vi "Remove Sink.vi"(8 "error in (no error)":errorcluster, 9 "Remove All (F)":bool, 10 "Sink Name":string, 11 "Event Source in":refnum<class "Event Source.lvclass">) -> (0 "error out":errorcluster, 3 "Event Source out":refnum<class "Event Source.lvclass">)   [LabVIEW 2016, in "Event Source.lvlib" / "Event Source.lvclass"]
doc: "Stops and removes a sink actor as specified by his name. Can remove all the sinks if the \"Remove All (F)\" is set to true"
uses:
  Event Source.lvclass
  Event Source.lvclass/Event Source.ctl
  Sink Details.ctl
  <vilib>/ActorFramework/Message Enqueuer/Message Enqueuer.lvclass
  <vilib>/ActorFramework/Message Enqueuer/Message Enqueuer.lvclass/Message Enqueuer.ctl
  <vilib>/ActorFramework/Message Enqueuer/Enqueue.vi
  <vilib>/ActorFramework/Stop Msg/Stop Msg.lvclass
  C:/Program Files (x86)/National Instruments/LabVIEW 2016/vi.lib/ActorFramework/Message/Message.lvclass
  <vilib>/Utility/LVClass/Get LV Class Name.vi
  <resource>/AFDebug/Generate Trace for Message.vi
  <vilib>/ActorFramework/Message Priority Queue/Priority Enqueue.vi
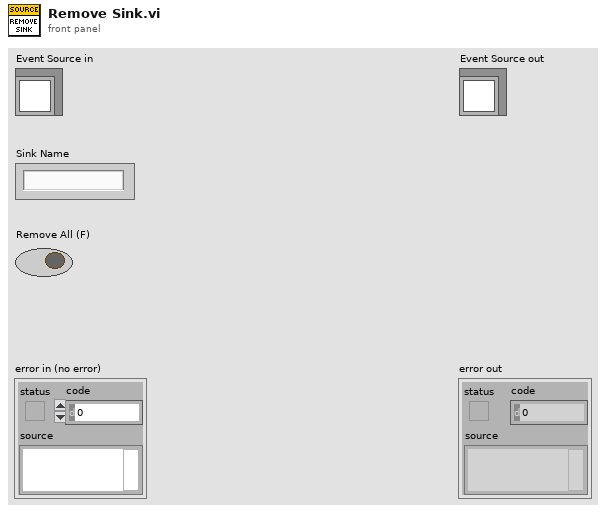
[diagram p1: front panel]
types:
  T1 = typedef "Event Source.lvlib/Event Source.lvclass/Sink Details.ctl" = cluster{"Exclude From Broadcast":bool, "Receive Only":bool, "Paused":bool, "Sink Enqueuer":refnum<class "Message Enqueuer.lvclass">}
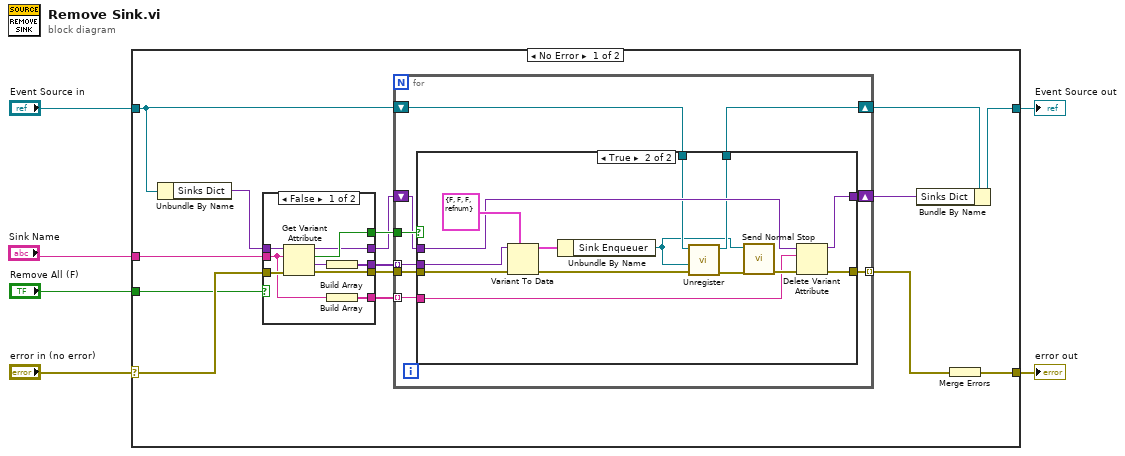
[diagram p0: block diagram]
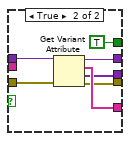
[diagram p3: hidden frame]
diagram:
  n1 = case shown="No Error" "error in (no error)" {
    selector: "error in (no error)" -> [w19 w65]
    tunnel: [w7 w65] -> w5
    tunnel: [w12 w64] -> w3
    tunnel: "Event Source in" -> [w14 w64]
    tunnel: "Sink Name" -> [w16 _]
    tunnel: "Remove All (F)" -> [w8 _]
    frame No Error {
      n2 = Unbundle By Name(w14) -> ("Sinks Dict"=w21:variant)
      n3 = case shown="False" w8 {
        tunnel: w21 -> [w56 w62]
        tunnel: [w55 TRUE] -> w20
        tunnel: w19 -> [w54 w63]
        tunnel: [w53 w59] -> w18
        tunnel: [w52 w60] -> w17
        tunnel: w16 -> [w51 _]
        tunnel: [w48 w58] -> w10
        tunnel: [w50 w61] -> w9
        frame False {
          n4 = Get Variant Attribute(Variant=w56, name=w51, error in=w54) -> (duplicate Variant=w53:variant, found=w55:bool, value=w49:variant, error out=w52:errorcluster)  [unwired: 1 in]
          n5 = Build Array(w49) -> (w48:variant[])
          n6 = Build Array(w51) -> (w50:string[])
        }
        frame True {
          n7 = Get Variant Attribute(Variant=w62, error in=w63) -> (duplicate Variant=w59:variant, names=w61:string[], values=w58:variant[], error out=w60:errorcluster)  [unwired: 2 in]
        }
      }
      n8 = for {
        tunnel: w20 -> [w30]
        tunnel: w10 -> [w23] mode=indexing
        tunnel: w9 -> [w22] mode=indexing
        shift-right: [w24] -> w11
        shift-left: w18 -> [w29]
        shift-right: [w25] -> w13
        shift-left: w14 -> [w26]
        tunnel: w17 -> [w28]
        tunnel: [w27] -> w15 mode=indexing
        n9 = case shown="True" w30 {
          tunnel: w29 -> [w31 w44]
          tunnel: w28 -> [w33 w47]
          tunnel: w22 -> [_ w43]
          tunnel: [w33 w42] -> w27
          tunnel: w26 -> [w32 w40]
          tunnel: [w32 w39] -> w25
          tunnel: [w31 w36] -> w24
          tunnel: w23 -> [_ w35]
          frame False {
          }
          frame True {
            n10 = Variant To Data(error in=w47, type=T1 {"Exclude From Broadcast"=FALSE, "Receive Only"=FALSE, "Paused"=FALSE, "Sink Enqueuer"=refnum} ("Actor's Enqueuer"), Variant=w35) -> (data=w37:T1, error out=w41:errorcluster)
            n11 = Unbundle By Name(w37) -> ("Sink Enqueuer"=w34:refnum<class "Message Enqueuer.lvclass">)
            n12 = call "Unregister.vi"("Error In"=w41, "Registrant Enq"=w34, "Event Source In"=w40) -> ("Error Out"=w38:errorcluster, "Event Source Out"=w39:refnum<class "Event Source.lvclass">)  [unwired: 7 in]
            n13 = call <vilib>:"Send Normal Stop.vi"("error in (no error)"=w38, "Message Enqueuer"=w34) -> ("error out"=w45:errorcluster)  [unwired: 9 in]
            n14 = Delete Variant Attribute(4:w45, 6:w43, 7:w44) -> (0:w42:errorcluster, 3:w36:variant)  [unwired: 1 out]
          }
        }
      }
      n15 = Bundle By Name(cluster=w13, "Sinks Dict"=w11) -> (w12:refnum<class "Event Source.lvclass">)
      n16 = Merge Errors(w15) -> (w7:errorcluster)
    }
    frame Error {
    }
  }
  "error out" <- w5
  "Event Source out" <- w3
